vi "Stop Core.vi"(10 "final error code":i32, 11 "Engine in":refnum<class "Engine.lvclass">) -> (3 "Engine out":refnum<class "Engine.lvclass">)   [LabVIEW 2023, in "Engine.lvlib" / "Engine.lvclass"]
uses:
  Library/Engine.lvclass
  builds/Framework/Panel Manager.lvlibp/Library/Panel Actor.lvclass
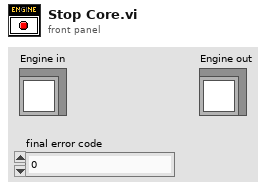
[diagram p1: front panel]
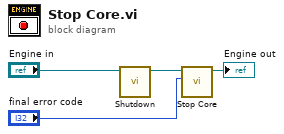
[diagram p0: block diagram]
diagram:
  n1 = call-dynamic "Shutdown.vi"("Engine in"="Engine in") -> ("Engine out"=w1:refnum<class "Engine.lvclass">)  [unwired: 9 in, 1 out]
  n2 = call-parent "Stop Core.vi"("final error code"="final error code", "Actor in"=w1) -> ("Actor out"=→"Engine out":refnum<class "Engine.lvclass">)  [unwired: 9 in]
